vi "0254-read-reference.vi"(10 "Channel Selction":i32, 11 "VISA Refnum in":refnum<visa-resource-name>) -> (0 "error out":errorcluster, 2 "PV":dbl, 3 "VISA Refnum out":refnum<visa-resource-name>)   [LabVIEW 2015]
uses:
  <vilib>/Instr/_visa.llb/VISA Configure Serial Port (Instr).vi
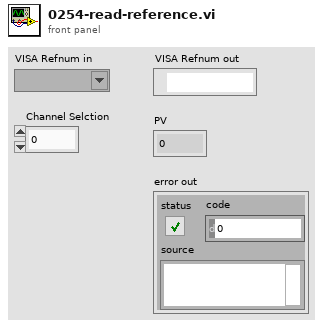
[diagram p1: front panel]
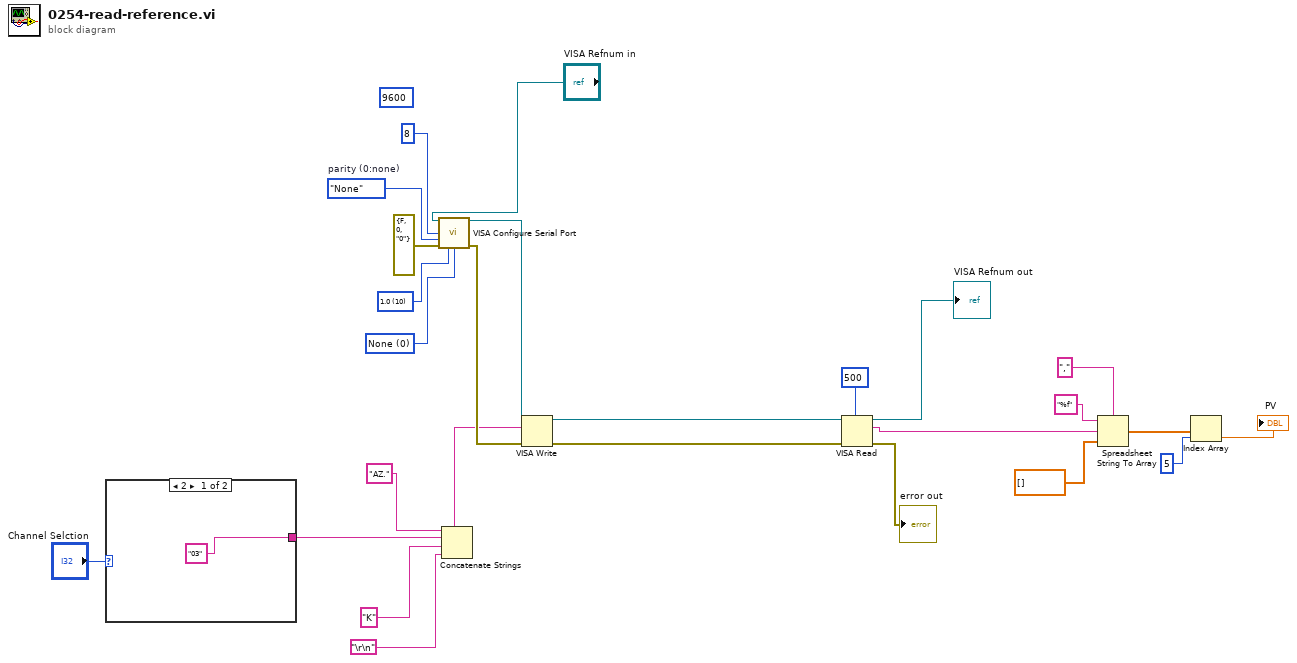
[diagram p0: block diagram]
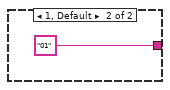
[diagram p2: hidden frame]
diagram:
  w16 = u16 0 items=["None", "XON/XOFF", "RTS/CTS", "XON/XOFF & RTS/CTS", "DTR/DSR", "XON/XOFF & DTR/DSR"] ("flow control (0:none)")
  w15 = u16 10 items=["1.0"=10, "1.5"=15, "2.0"=20] ("stop bits (10: 1 bit)")
  w14 = enum16{"None", "Odd", "Even", "Mark", "Space"}."None"  # parity (0:none)
  (unwired) u32 9600 ("baud rate (9600)")
  n1 = case shown="2" "Channel Selction" {
    tunnel: ["03" "01"] -> w23
    frame 2 {
    }
    frame 1, Default {
    }
  }
  n2 = call-poly "VISA Configure Serial Port"("VISA resource name"="VISA Refnum in", "data bits (8)"=u16 8, "parity (0:none)"=w14, "error in (no error)"=errorcluster {"status"=FALSE, "code"=0, "source"="0"}, "stop bits (10: 1 bit)"=w15, "flow control (0:none)"=w16) -> ("VISA resource name out"=w18:refnum<visa-resource-name>, "error out"=w25:errorcluster)  [unwired: 8 in]
  n3 = Concatenate Strings("AZ." ("string"), w23, "K" ("string"), "\r\n") -> (w8:string)
  n4 = VISA Write(VISA resource name=w18, write buffer=w8, error in (no error)=w25) -> (VISA resource name out=w10:refnum<visa-resource-name>, error out=w12:errorcluster)  [unwired: 1 out]
  n5 = VISA Read(VISA resource name=w10, byte count=u32 500, error in (no error)=w12) -> (VISA resource name out=→"VISA Refnum out":refnum<visa-resource-name>, read buffer=w7:string, error out=→"error out":errorcluster)  [unwired: 1 out]
  n6 = Spreadsheet String To Array(delimiter (Tab)=",", format string="%f", spreadsheet string=w7, array type (2D Dbl)=dbl[] []) -> (array=w1:dbl[])
  n7 = Index Array(array=w1, index=5) -> (element=→"PV":dbl)
